vi "Voorbeeld_Zoek_Getal_Array.vi"() -> ()   [LabVIEW 2019]
panel:
  out "Array 2":i32[](array[numeric])
  out "Aantal":i32
  in  "Getal":i32
  in  "ZoekArray":i32[](array[numeric])
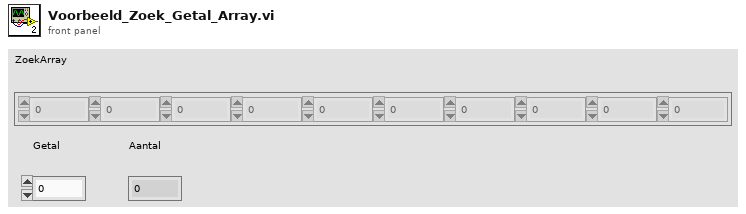
[diagram p1: front panel]
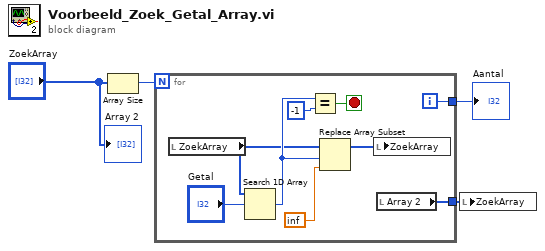
[diagram p0: block diagram]
diagram:
  n1 = Array Size(array="ZoekArray") -> (size(s)=w4:i32)
  n2 = for {
    N: w4 -> [_]
    tunnel: [w12] -> w2
    tunnel: [w5] -> w1
    i -> [w12]
    stop <- w10 stop-if-true
    n3 = local read "ZoekArray"() -> (w6:i32[])
    n4 = Search 1D Array(1D array=w6, element="Getal") -> (index of element=w8:i32)  [unwired: 1 in]
    n5 = Equal?(x=w8, y=-1) -> (x = y?=w10:bool)
    n6 = Replace Array Subset(array=w6, new element=inf, index=w8) -> (w7:i32[])
    n7 = local write "ZoekArray"(w7) -> ()
    n8 = local read "Array 2"() -> (w5:i32[])
  }
  "Aantal" <- w2
  n9 = local write "ZoekArray"(w1) -> ()
  "Array 2" <- "ZoekArray"
